vi "Car Wash.vi"() -> ()   [LabVIEW 2020]
uses:
  Controls/Car Wash Indicators.ctl
  Controls/Wash Options.ctl
  Controls/Car Wash References.ctl
  Controls/Wash Steps Selected-Update Display Message.ctl
  Controls/Timer Controls.ctl
  Support/Enqueue Message (Single).vi
  <vilib>/Utility/error.llb/Error Cluster From Error Code.vi
  <vilib>/ErrorRing/Error Ring.xnode
  Support/Message Queue.lvlib
panel:
  in  "Start":bool
  out "Elapsed Time":dbl format="%0.2f"
  in  "stop":bool
  out "Wash Entry":bool
  in  "Wash Options":T1
  in  "Car Position Slider":u8(slide) max=3 scale=0.0..4.0
  out "Car Wash Indicators":T2
  # "Entry Console"
  # "Car Wash Display"
  # "Car Position Simulation"
  # "Pre-Soak\nH-P Wash\nL-P Wax\nSpot Free Rinse"
  # "Underbody Wash\nBug Remover"
  # "Tire Shine\nAir Dry"
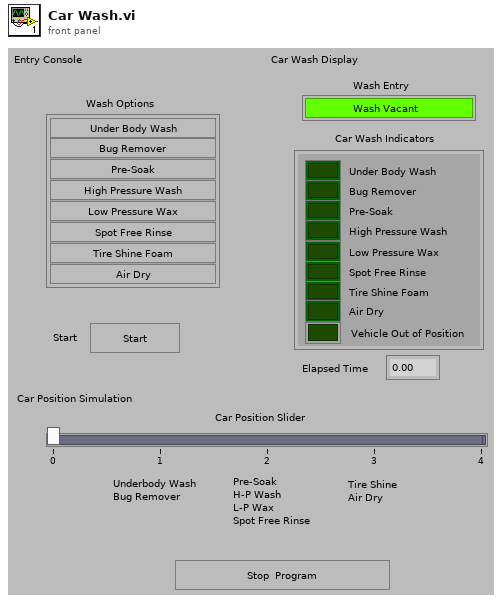
[diagram p1: front panel]
types:
  T1 = typedef "Wash Options.ctl" = cluster{"Underbody Wash":bool, "Bug Remover":bool, "Pre-Soak":bool, "High Pressure Wash":bool, "Low Pressure Wax":bool, "Spot Free Rinse":bool, "Tire Shine Foam":bool, "Air Dry":bool}
  T2 = typedef "Car Wash Indicators.ctl" = cluster{"Under Body Wash":bool, "Bug Remover":bool, "Pre-Soak":bool, "High Pressure Wash":bool, "Low Pressure Wax":bool, "Spot Free Rinse":bool, "Tire Shine Foam":bool, "Air Dry":bool, "Vehicle Out of Position":bool}
  T3 = typedef "Car Wash References.ctl" = cluster{"Car Wash Indicators Ref":refnum<vi>, "Wash Options Ref":refnum<vi>, "Car Position Slider Ref":refnum<vi>, "Elapsed Time Ref":refnum<vi>, "Wash Entry Ref":refnum<vi>, "Start Ref":refnum<vi>}
  T4 = typedef "Message Queue.lvlib/All Message Queues.ctl" = cluster{"UI":refnum<queue>}
  T5 = typedef "Wash Steps Selected-Update Display Message.ctl" = cluster{"Wash Steps Selected":cluster{"Wash Step":string, "Step Time":i32, "Station":string}[], "Update Display Message":string}
  T6 = enum8{"Enabled", "Disabled", "Disabled and Grayed Out"}
  T7 = typedef "Timer Controls.ctl" = enum16{"Reset", "Start", "Stop"}
  T8 = cluster{"Wash Step":string, "Step Time":i32, "Station":string}[]
  T9 = cluster{"Wash Step":string, "Step Time":i32, "Station":string}
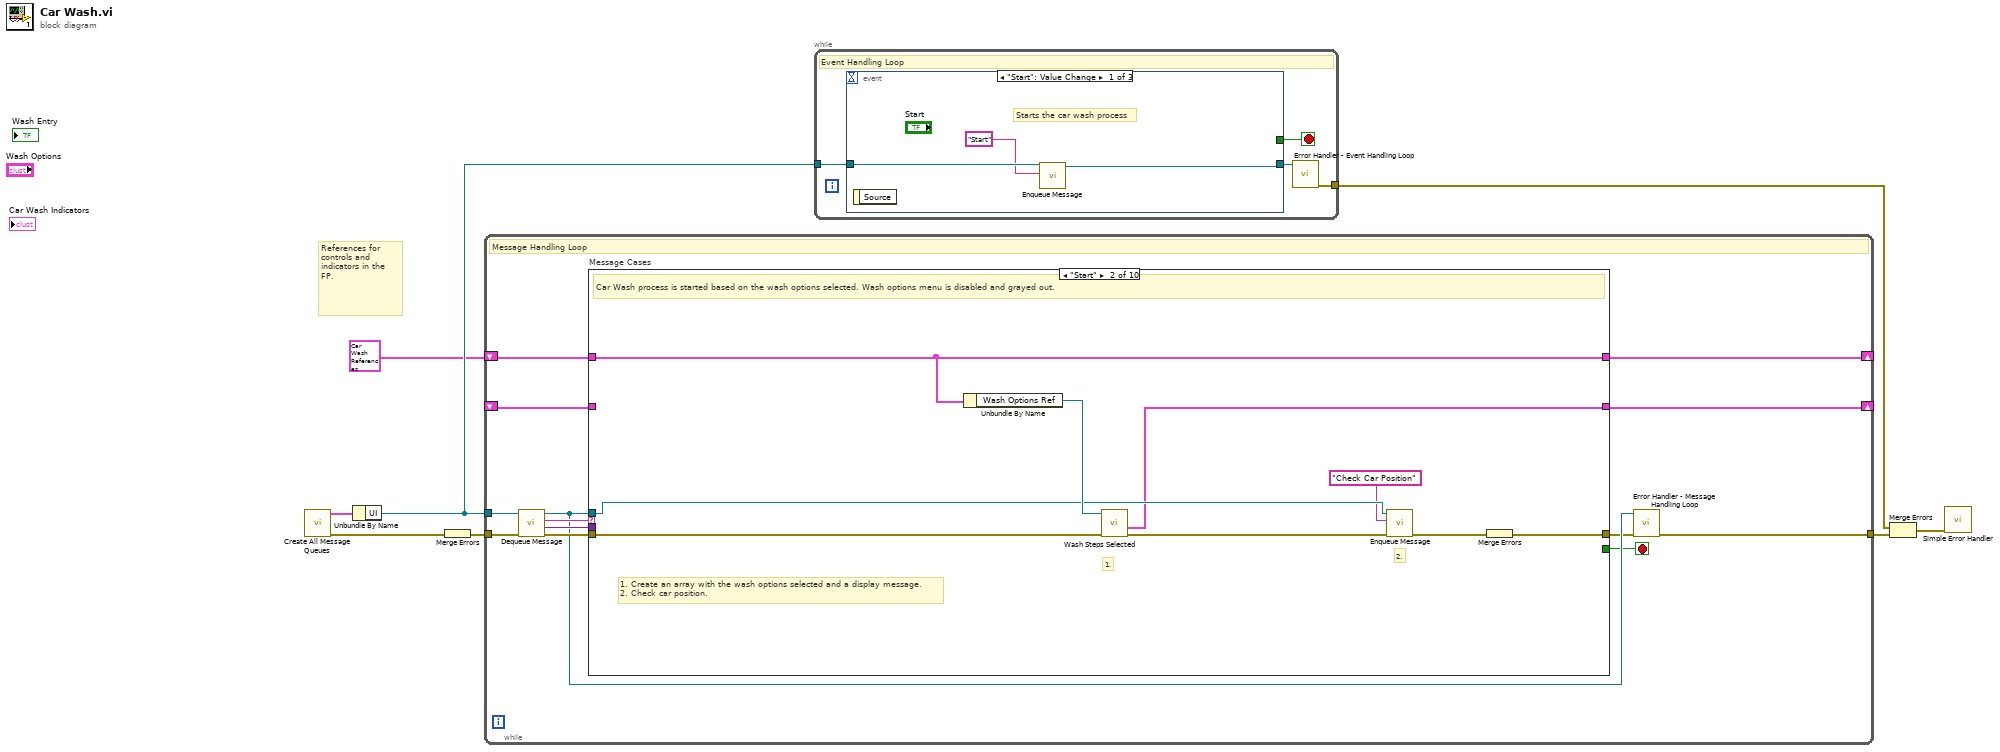
[diagram p0: block diagram]
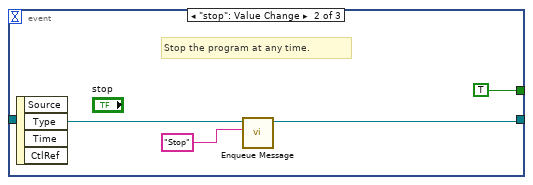
[diagram p2: hidden frame]
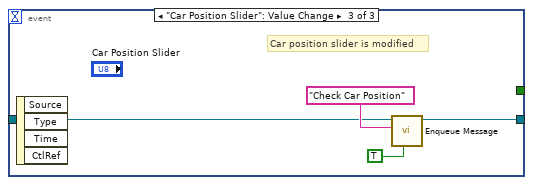
[diagram p3: hidden frame]
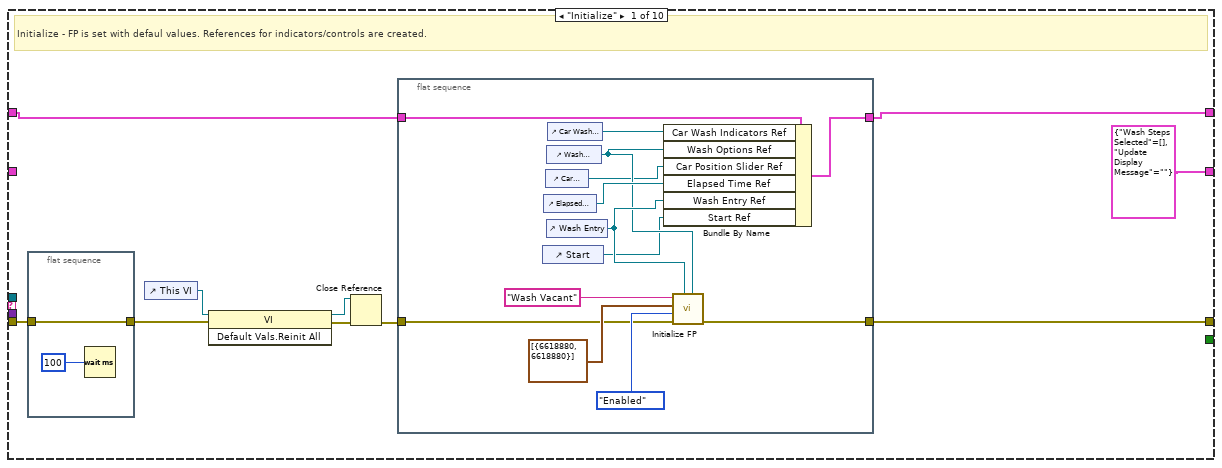
[diagram p4: hidden frame]
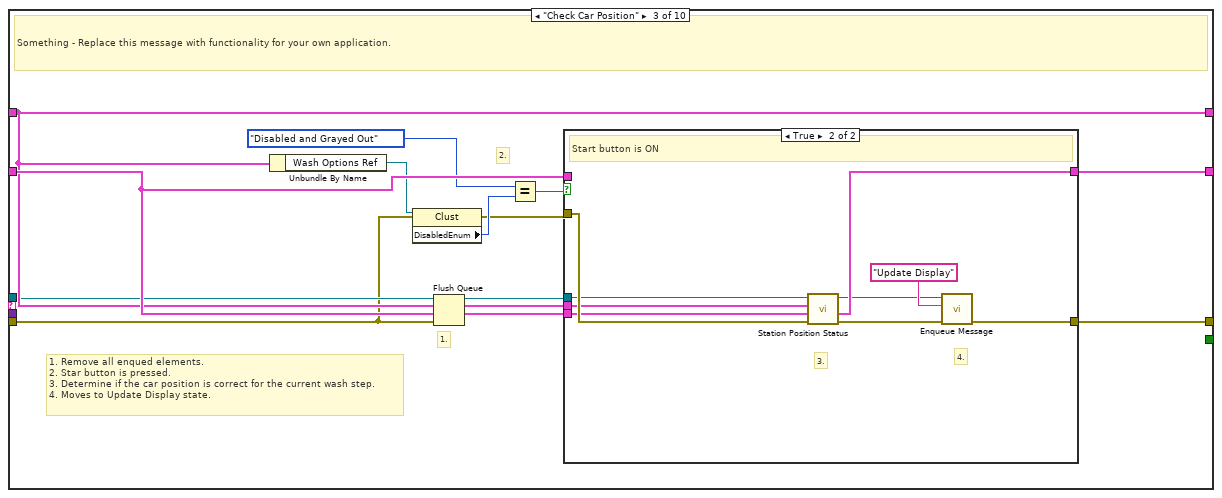
[diagram p5: hidden frame]
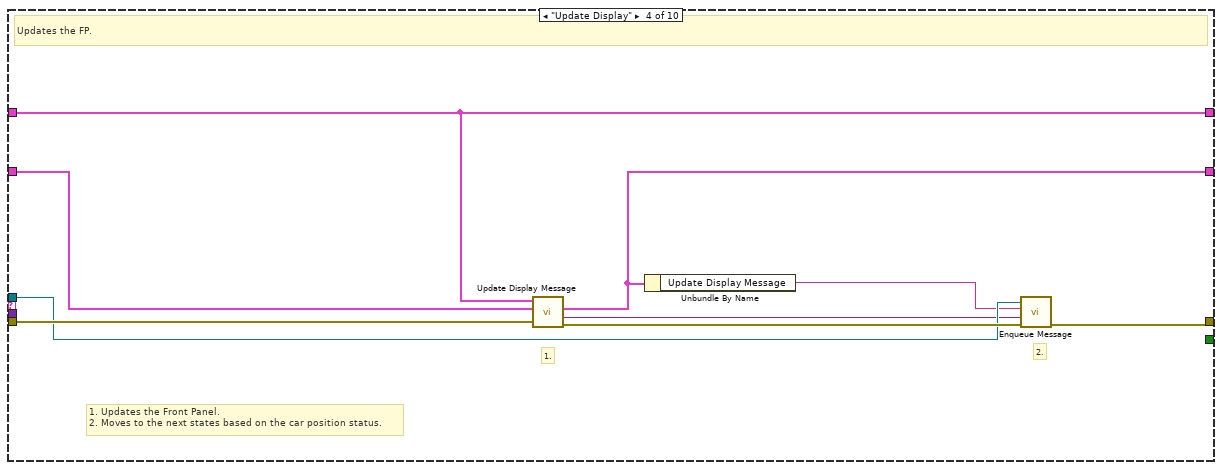
[diagram p7: hidden frame]
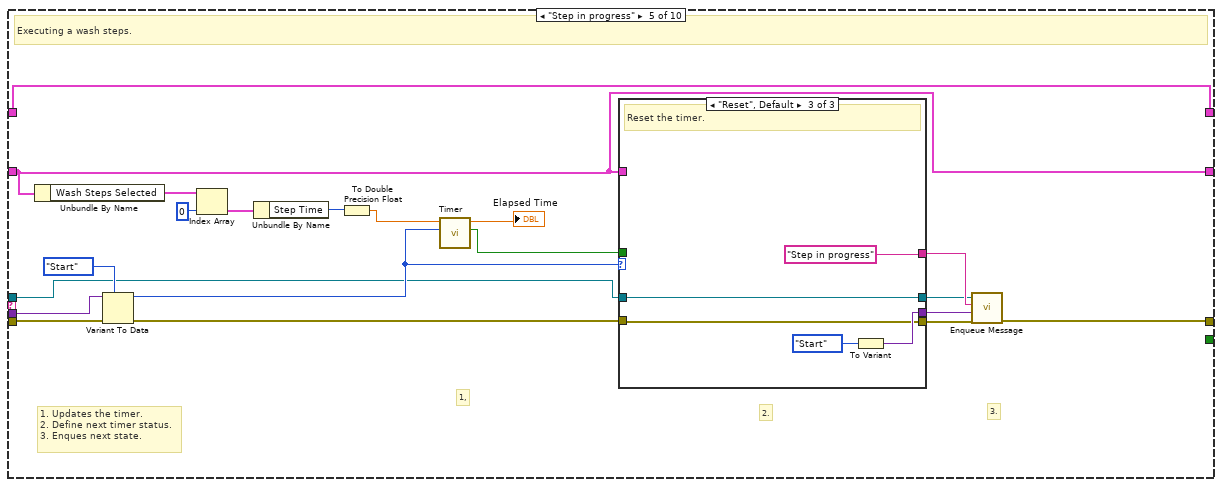
[diagram p8: hidden frame]
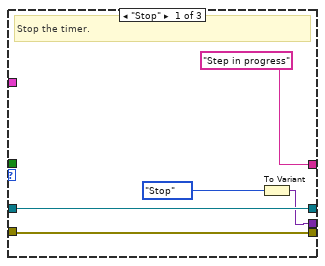
[diagram p9: hidden frame]
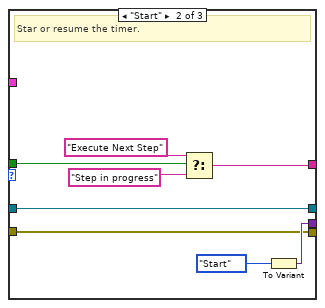
[diagram p10: hidden frame]
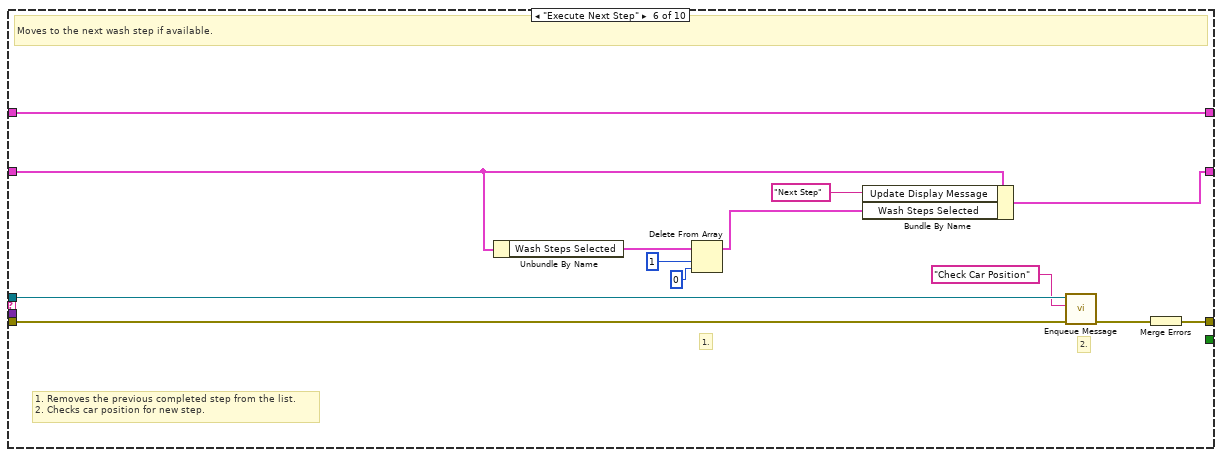
[diagram p11: hidden frame]
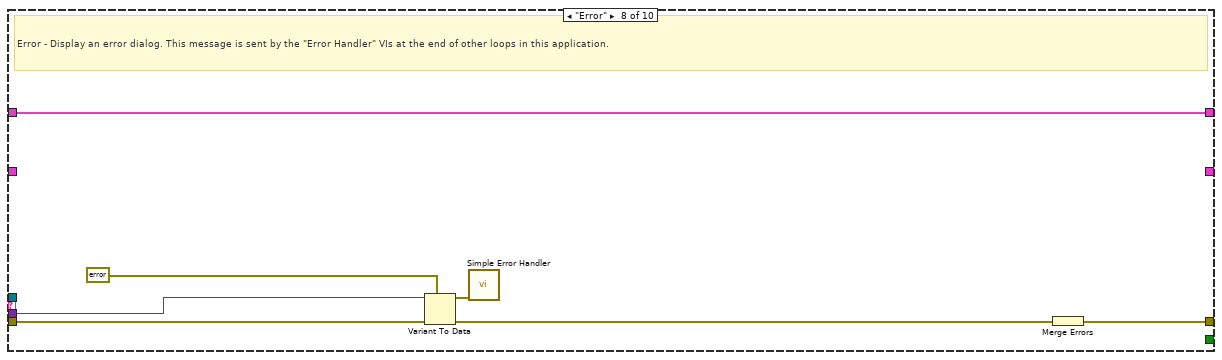
[diagram p13: hidden frame]
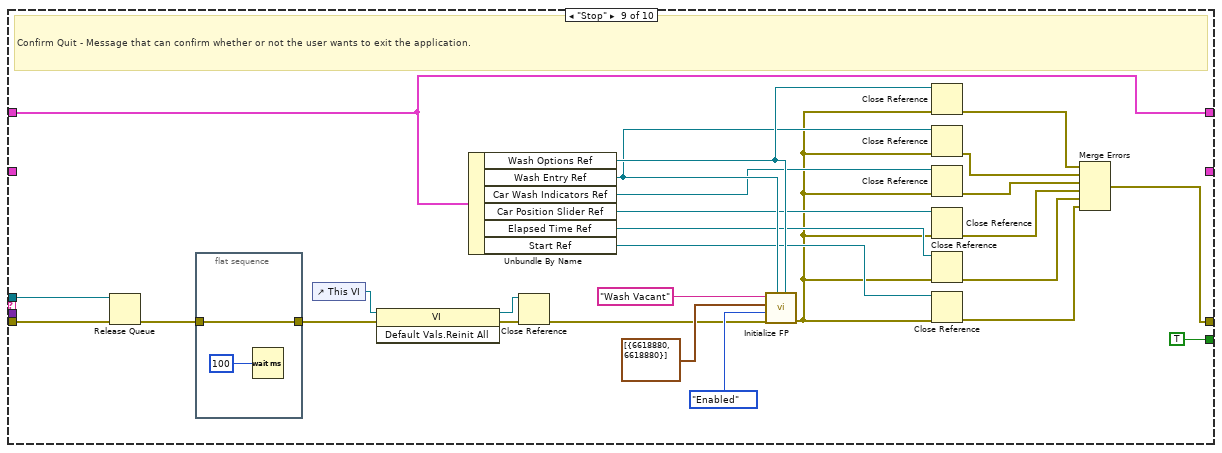
[diagram p14: hidden frame]
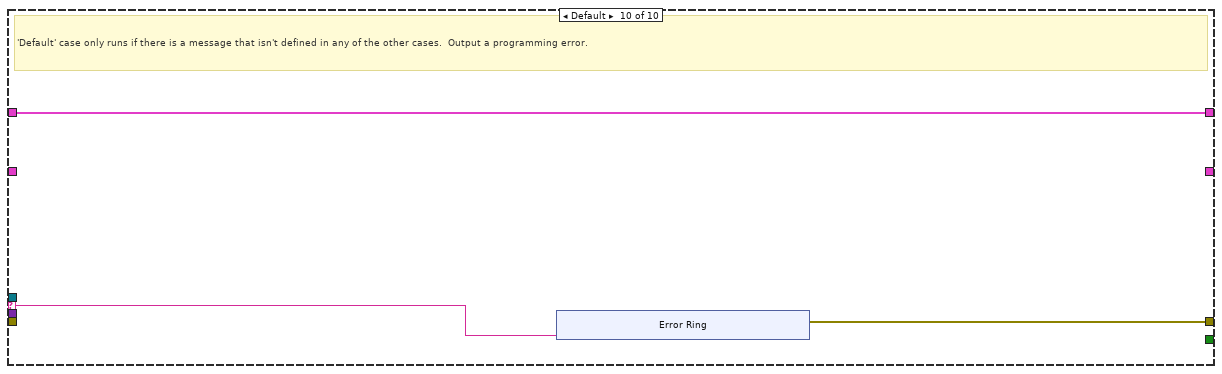
[diagram p15: hidden frame]
diagram:
  # "References for controls and indicators in the FP."
  n1 = call "Create All Message Queues.vi"() -> ("error out"=w8:errorcluster, "Message Queues out"=w7:T4)  [unwired: 10 in]
  n2 = Unbundle By Name(w7) -> ("UI"=w5:refnum<queue>)
  n3 = Merge Errors(w8) -> (w3:errorcluster)
  n4 = while {
    tunnel: w5 -> [w15]
    shift-right: [w20] -> _
    shift-left: T3 {"Car Wash Indicators Ref"=refnum, "Wash Options Ref"=refnum, "Car Position Slider Ref"=refnum, "Elapsed Time Ref"=refnum, "Wash Entry Ref"=refnum, "Start Ref"=refnum} ("Data Cluster") -> [w21]
    tunnel: w3 -> [w19]
    tunnel: [w13] -> w6
    shift-right: [w10] -> _
    shift-left: _ -> [w9]
    stop <- w11 stop-if-true
    # "Message Handling Loop"
    n5 = call "Dequeue Message.vi"("error in (no error)"=w19, "Message Queue"=w15) -> ("error out"=w18:errorcluster, "Message Data"=w16:variant, "Message"=w17:string, "dup Message Queue"=w14:refnum<queue>)  [unwired: 6 in]
    n6 = case "Message Cases" shown="\"Start\"" w17 {
      selector: w17 -> [_ _ _ _ _ _ _ _ _ w177]
      tunnel: w14 -> [_ w50 w57 w82 w91 w134 _ _ w173 _]
      tunnel: w18 -> [w26 w53 w56 w86 w100 w126 w138 w147 w172 _]
      tunnel: [w27 w55 w67 w83 w92 w136 w138 w141 w149 w178] -> w12
      tunnel: w21 -> [w31 w54 w64 w85 w106 w137 w140 w146 w148 w179]
      tunnel: [w29 w54 w64 w85 w106 w137 w140 w146 w148 w179] -> w20
      tunnel: w16 -> [_ _ _ _ w101 _ _ w145 _ _]
      tunnel: [_ _ _ _ _ _ _ _ TRUE _] -> w11
      tunnel: [T5 {"Wash Steps Selected"=[], "Update Display Message"=""} ("Wash Steps Selected-Update Display Message") w48 w66 w79 w89 w125 w139 _ _ _] -> w10
      tunnel: w9 -> [_ _ w65 w80 w89 w129 w139 _ _ _]
      frame "Initialize" {
        # "Initialize - FP is set with defaul values. References for indicators/controls are created."
        n7 = flat-sequence {
          tunnel: w26 -> [w32]
          tunnel: [w32] -> w25
          frame #0 {
            n8 = Wait (ms)(milliseconds to wait=u32 100) -> ()  [unwired: 1 out]
          }
        }
        n9 = control-ref of="This VI"() -> (w28:refnum<vi>)
        n10 = invoke class="VI" method="Default Vals.Reinit All"(reference=w28, error in=w25) -> (reference out=w22:refnum<vi>, error out=w23:errorcluster)  [unwired: 1 in, 1 out]
        n11 = Close Reference(reference=w22, error in (no error)=w23) -> (error out=w24:errorcluster)
        n12 = flat-sequence {
          tunnel: w31 -> [w46]
          tunnel: [w37] -> w29
          tunnel: w24 -> [w36]
          tunnel: [w35] -> w27
          frame #0 {
            n13 = control-ref of="Start"() -> (w39:refnum<vi>)
            n14 = control-ref of="Elapsed Time"() -> (w45:refnum<vi>)
            n15 = control-ref of="Car Position Slider"() -> (w34:refnum<vi>)
            n16 = control-ref of="Wash Options"() -> (w40:refnum<vi>)
            n17 = control-ref of="Wash Entry"() -> (w41:refnum<vi>)
            n18 = control-ref of="Car Wash Indicators"() -> (w44:refnum<vi>)
            n19 = Bundle By Name(cluster=w46, "Car Wash Indicators Ref"=w44, "Wash Options Ref"=w40, "Car Position Slider Ref"=w34, "Elapsed Time Ref"=w45, "Wash Entry Ref"=w41, "Start Ref"=w39) -> (w37:T3)
            n20 = call "Initialize FP.vi"("Wash Options Ref"=w40, "Wash Entry Ref"=w41, "error in"=w36, "Enable\\Disable Wash Options"=T6."Enabled" ("Enable\\Disable Wash Options"), "Wash In Progress Color"=cluster{u32, u32}[] [{6618880, 6618880}], "Wash In Progress Text"="Wash Vacant") -> ("error out"=w35:errorcluster)  [unwired: 5 in]
          }
        }
      }
      frame "Start" {
        # "1. Create an array with the wash options selected and a display message.\n2. Check car position."
        # "2."
        # "1."
        # "Car Wash process is started based on the wash options selected. Wash options menu is disabled and grayed out."
        n21 = Unbundle By Name(w54) -> ("Wash Options Ref"=w52:refnum<vi>)
        n22 = call "Wash Steps Selected.vi"("error in (no error)"=w53, "Wash Options Ref"=w52) -> ("error out"=w47:errorcluster, "Wash Steps Selected-Update Display Message"=w48:T5)  [unwired: 8 in]
        n23 = call-poly "Enqueue Message.vi"("error in (no error)"=w47, "Message"="Check Car Position", "Message Queue"=w50) -> ("error out"=w51:errorcluster)  [unwired: 7 in, 1 out]
        n24 = Merge Errors(w51) -> (w55:errorcluster)
      }
      frame "Check Car Position" {
        # "1. Remove all enqued elements.\n2. Star button is pressed.\n3. Determine if the car position is correct for the current wash step. \n4. Moves to Update Display state."
        # "1."
        # "2."
        # "Something - Replace this message with functionality for your own application."
        n25 = Unbundle By Name(w64) -> ("Wash Options Ref"=w63:refnum<vi>)
        n26 = property class="Clust"(reference=w63, error in=w56) -> (error out=w59:errorcluster, "DisabledEnum"=w61:T6)  [unwired: 1 out]
        n27 = Flush Queue(queue=w57, error in (no error)=w56) -> (queue out=w58:refnum<queue>)  [unwired: 2 out]
        n28 = Equal?(x=T6."Disabled and Grayed Out", y=w61) -> (x = y?=w62:bool)
        n29 = case shown="True" w62 {
          tunnel: [w68 w74] -> w67
          tunnel: w58 -> [_ w70]
          tunnel: w64 -> [_ w71]
          tunnel: w65 -> [_ w72]
          tunnel: [w69 w75] -> w66
          tunnel: w65 -> [w69 _]
          tunnel: w59 -> [w68 w73]
          frame False {
            # "Start button is OFF"
          }
          frame True {
            # "4."
            # "3."
            # "Start button is ON"
            n30 = call "Station Position Status.vi"("error in (no error)"=w73, "Wash Steps Selected-Update Display Message"=w72, "Car Wash References"=w71) -> ("error out"=w77:errorcluster, "Message Out"=w75:T5)  [unwired: 5 in]
            n31 = call-poly "Enqueue Message.vi"("error in (no error)"=w77, "Message"="Update Display", "Message Queue"=w70) -> ("error out"=w74:errorcluster)  [unwired: 7 in, 1 out]
          }
        }
      }
      frame "Update Display" {
        # "1. Updates the Front Panel.\n2. Moves to the next states based on the car position status."
        # "2."
        # "1."
        # "Updates the FP."
        n32 = call "Update Display Message.vi"("error in (no error)"=w86, "Wash Steps Selected-Update Display Message In"=w80, "Data Cluster"=w85) -> ("error out"=w84:errorcluster, "Step in progress timer control"=w78:variant, "Wash Steps Selected-Update Display Message Out"=w79:T5)  [unwired: 6 in]
        n33 = Unbundle By Name(w79) -> ("Update Display Message"=w81:string)
        n34 = call-poly "Enqueue Message.vi"("error in (no error)"=w84, "Message Data"=w78, "Message"=w81, "Message Queue"=w82) -> ("error out"=w83:errorcluster)  [unwired: 6 in, 1 out]
      }
      frame "Step in progress" {
        # "1. Updates the timer.\n2. Define next timer status.\n3. Enques next state."
        # "3."
        # "2."
        # "1,"
        # "Executing a wash steps."
        n35 = Unbundle By Name(w89) -> ("Wash Steps Selected"=w105:T8)
        n36 = Variant To Data(error in=w100, type=Timer_Controls."Start", Variant=w101) -> (data=w98:T7, error out=w99:errorcluster)
        n37 = Index Array(array=w105, index=0) -> (element=w103:T9)
        n38 = Unbundle By Name(w103) -> ("Step Time"=w102:i32)
        n39 = To Double Precision Float(number=w102) -> (double precision float=w88:dbl)
        n40 = call "Timer.vi"("Timer Control"=w98, "Time Target"=w88) -> ("Time completed?"=w97:bool, "Elapsed Time"=→"Elapsed Time":dbl)  [unwired: 8 in]
        n41 = case shown="\"Reset\", Default" w98 {
          tunnel: w91 -> [w110 w114 w123]
          tunnel: w99 -> [w111 w115 w121]
          tunnel: [w111 w115 w121] -> w87
          tunnel: w97 -> [_ w117 _]
          tunnel: [w108 w116 w122] -> w94
          tunnel: ["Step in progress" ("Message") w113 "Step in progress" ("Message")] -> w93
          tunnel: [w110 w114 w123] -> w90
          tunnel: w89 -> [_ _ _]
          frame "Stop" {
            # "Stop the timer."
            n42 = To Variant(anything=Timer_Controls."Stop" ("Enum")) -> (Variant=w108:variant)
          }
          frame "Start" {
            # "Star or resume the timer."
            n43 = Select(t="Execute Next Step" ("Message"), s=w117, f="Step in progress" ("Message")) -> (s? t:f=w113:string)
            n44 = To Variant(anything=Timer_Controls."Start" ("Enum")) -> (Variant=w116:variant)
          }
          frame "Reset", Default {
            # "Reset the timer."
            n45 = To Variant(anything=Timer_Controls."Start" ("Enum")) -> (Variant=w122:variant)
          }
        }
        n46 = call-poly "Enqueue Message.vi"("error in (no error)"=w87, "Message Data"=w94, "Message"=w93, "Message Queue"=w90) -> ("error out"=w92:errorcluster)  [unwired: 6 in, 1 out]
      }
      frame "Execute Next Step" {
        # "1. Removes the previous completed step from the list.\n2. Checks car position for new step."
        # "2."
        # "1."
        # "Moves to the next wash step if available."
        n47 = Unbundle By Name(w129) -> ("Wash Steps Selected"=w127:T8)
        n48 = Delete From Array(array=w127, length=1, index=0) -> (array with subset deleted=w128:T8)  [unwired: 1 out]
        n49 = Bundle By Name(cluster=w129, "Update Display Message"="Next Step", "Wash Steps Selected"=w128) -> (w125:T5)
        n50 = call-poly "Enqueue Message.vi"("error in (no error)"=w126, "Message"="Check Car Position", "Message Queue"=w134) -> ("error out"=w135:errorcluster)  [unwired: 7 in, 1 out]
        n51 = Merge Errors(w135) -> (w136:errorcluster)
      }
      frame "Vehicle Out of Position" {
        # "Vehicle is Out of Position. Waiting for the right Car position."
      }
      frame "Error" {
        # "Error - Display an error dialog. This message is sent by the \"Error Handler\" VIs at the end of other loops in this application."
        n52 = Variant To Data(error in=w147, type=errorcluster {"status"=FALSE, "code"=0, "source"=""} ("error constant"), Variant=w145) -> (data=w143:errorcluster, error out=w142:errorcluster)
        n53 = call <vilib>:"Simple Error Handler.vi"("error in (no error)"=w143) -> ()  [unwired: 4 in, 5 out]
        n54 = Merge Errors(w142) -> (w141:errorcluster)
      }
      frame "Stop" {
        # "Confirm Quit - Message that can confirm whether or not the user wants to exit the application."
        n55 = Release Queue(queue=w173, error in (no error)=w172) -> (error out=w168:errorcluster)  [unwired: 1 in, 2 out]
        n56 = flat-sequence {
          tunnel: w168 -> [w175]
          tunnel: [w175] -> w167
          frame #0 {
            n57 = Wait (ms)(milliseconds to wait=u32 100) -> ()  [unwired: 1 out]
          }
        }
        n58 = control-ref of="This VI"() -> (w171:refnum<vi>)
        n59 = invoke class="VI" method="Default Vals.Reinit All"(reference=w171, error in=w167) -> (reference out=w169:refnum<vi>, error out=w170:errorcluster)  [unwired: 1 in, 1 out]
        n60 = Unbundle By Name(w148) -> ("Wash Options Ref"=w162:refnum<vi>, "Wash Entry Ref"=w161:refnum<vi>, "Car Wash Indicators Ref"=w160:refnum<vi>, "Car Position Slider Ref"=w159:refnum<vi>, "Elapsed Time Ref"=w158:refnum<vi>, "Start Ref"=w157:refnum<vi>)
        n61 = Close Reference(reference=w169, error in (no error)=w170) -> (error out=w163:errorcluster)
        n62 = call "Initialize FP.vi"("Wash Options Ref"=w162, "Wash Entry Ref"=w161, "error in"=w163, "Enable\\Disable Wash Options"=T6."Enabled" ("Enable\\Disable Wash Options"), "Wash In Progress Color"=cluster{u32, u32}[] [{6618880, 6618880}], "Wash In Progress Text"="Wash Vacant") -> ("error out"=w156:errorcluster)  [unwired: 5 in]
        n63 = Close Reference(reference=w162, error in (no error)=w156) -> (error out=w155:errorcluster)
        n64 = Close Reference(reference=w161, error in (no error)=w156) -> (error out=w154:errorcluster)
        n65 = Close Reference(reference=w160, error in (no error)=w156) -> (error out=w153:errorcluster)
        n66 = Close Reference(reference=w159, error in (no error)=w156) -> (error out=w152:errorcluster)
        n67 = Close Reference(reference=w158, error in (no error)=w156) -> (error out=w151:errorcluster)
        n68 = Close Reference(reference=w157, error in (no error)=w156) -> (error out=w150:errorcluster)
        n69 = Merge Errors(w155, w154, w153, w152, w151, w150) -> (w149:errorcluster)
      }
      frame Default {
        # "'Default' case only runs if there is a message that isn't defined in any of the other cases.  Output a programming error."
        n70 = xnode "Error Ring"("parameter 0"=w177) -> ("error out"=w178:errorcluster)
      }
    }
    n71 = call "Error Handler - Message Handling Loop.vi"("error in (no error)"=w12, "Message Queue"=w14) -> ("dup error in"=w13:errorcluster)  [unwired: 8 in, 1 out]
  }
  n72 = while {
    tunnel: w5 -> [w190]
    tunnel: [w187] -> w2
    stop <- w189 stop-if-true
    # "Event Handling Loop"
    n73 = event shown="[0] \"Start\": Value Change" {
      selector: _ -> [_ _ _]
      dyn-events: _ -> [_ _ _]
      timeout: _ -> [_ _ _]
      tunnel: [_ TRUE ("Discard?") _] -> w189
      tunnel: w190 -> [w193 w196 w199]
      tunnel: [w192 w195 w201] -> w188
      event "Start": Value Change {
        # "Starts the car wash process"
        n74 = event-data() -> ()  [unwired: 1 in, 1 out]
        n75 = call-poly "Enqueue Message.vi"("Message"="Start", "Message Queue"=w193) -> ("dup Message Queue"=w192:refnum<queue>)  [unwired: 8 in, 1 out]
      }
      event "stop": Value Change {
        # "Stop the program at any time."
        n76 = event-data() -> ()  [unwired: 1 in, 4 out]
        n77 = call-poly "Enqueue Message.vi"("Message"="Stop", "Message Queue"=w196) -> ("dup Message Queue"=w195:refnum<queue>)  [unwired: 8 in, 1 out]
      }
      event "Car Position Slider": Value Change {
        # "Car position slider is modified"
        n78 = event-data() -> ()  [unwired: 1 in, 4 out]
        n79 = call-poly "Enqueue Message.vi"("Priority Message? (F)"=TRUE, "Message"="Check Car Position", "Message Queue"=w199) -> ("dup Message Queue"=w201:refnum<queue>)  [unwired: 7 in, 1 out]
      }
    }
    n80 = call "Error Handler - Event Handling Loop.vi"("Message Queue"=w188) -> ("dup error in"=w187:errorcluster)  [unwired: 9 in, 1 out]
  }
  n81 = Merge Errors(w2, w6) -> (w1:errorcluster)
  n82 = call <vilib>:"Simple Error Handler.vi"("error in (no error)"=w1) -> ()  [unwired: 4 in, 5 out]
